vi "DK240 Read.vi"(3 "error in":errorcluster, 4 "Byte count":u32, 5 "Port":refnum<visa-resource-name>) -> (0 "error out":errorcluster, 1 "Received Bytes":u8[](array[numeric]))   [LabVIEW 2010]
doc: "Ce Vi lit le nombre de bytes indiqués du port série spécifié et les retourne sous forme de tableau."
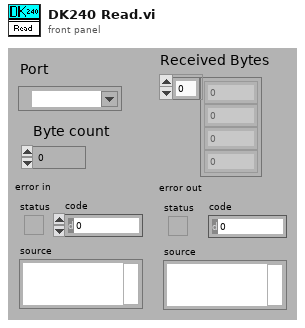
[diagram p1: front panel]
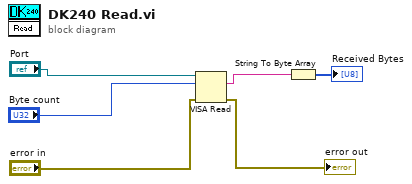
[diagram p0: block diagram]
diagram:
  n1 = VISA Read(VISA resource name="Port", byte count="Byte count", error in (no error)="error in") -> (read buffer=w3:string, error out=→"error out":errorcluster)  [unwired: 2 out]
  n2 = String To Byte Array(string=w3) -> (unsigned byte array=→"Received Bytes":u8[])
